vi "Set A-B Tovey.vi"(10 "A-B Tovey":refnum<class "Tovey 9150.lvclass">, 11 "Model in":refnum<class "Model.lvclass">) -> (3 "Model out":refnum<class "Model.lvclass">)   [LabVIEW 2015, in "Model.lvclass"]
uses:
  Model.lvclass
  TEI-9150/Tovey 9150.lvclass
  Model.lvclass/Model.ctl
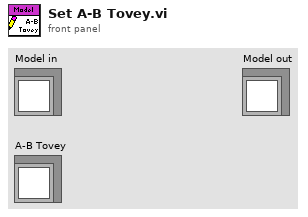
[diagram p1: front panel]
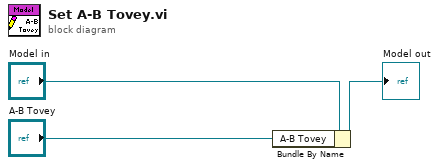
[diagram p0: block diagram]
diagram:
  n1 = Bundle By Name(cluster="Model in", "A-B Tovey"="A-B Tovey") -> (→"Model out":refnum<class "Model.lvclass">)
